vi "Sender.vi"() -> ()   [LabVIEW 2014]
uses:
  Global 1.vi
panel:
  out "Waveform Chart":dbl(graph)
  in  "Saving":bool
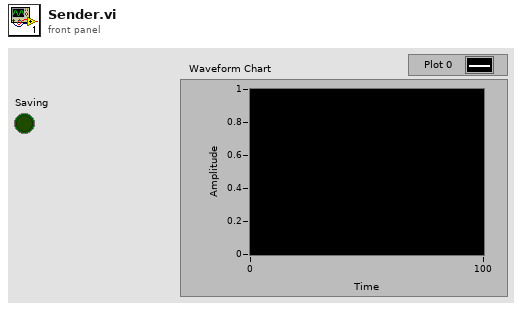
[diagram p1: front panel]
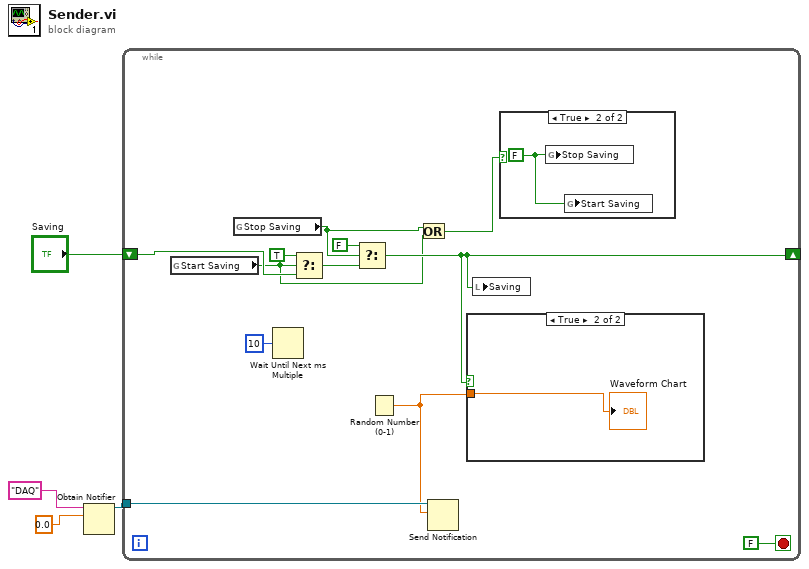
[diagram p0: block diagram]
diagram:
  n1 = Obtain Notifier(name (unnamed)="DAQ", notification data type=0.0) -> (notifier out=w3:refnum<notifier>)  [unwired: 2 in, 2 out]
  n2 = while {
    tunnel: w3 -> [w15]
    shift-right: [w8] -> _
    shift-left: "Saving" -> [w10]
    stop <- FALSE stop-if-true
    n3 = global read "Global 1.vi" "Start Saving"() -> (w6:bool)
    n4 = global read "Global 1.vi" "Stop Saving"() -> (w7:bool)
    n5 = Wait Until Next ms Multiple(millisecond multiple=u32 10) -> ()  [unwired: 1 out]
    n6 = Select(t=TRUE, s=w6, f=w10) -> (s? t:f=w12:bool)
    n7 = Select(t=FALSE, s=w7, f=w12) -> (s? t:f=w8:bool)
    n8 = Random Number (0-1)() -> (number: 0 to 1=w14:dbl)
    n9 = Or(x=w7, y=w6) -> (x .or. y?=w5:bool)
    n10 = Send Notification(notification=w14, notifier=w15) -> ()  [unwired: 1 in, 2 out]
    n11 = case shown="True" w8 {
      tunnel: w14 -> [_ w18]
      frame False {
      }
      frame True {
        "Waveform Chart" <- w18
      }
    }
    n12 = local write "Saving"(w8) -> ()
    n13 = case shown="True" w5 {
      frame False {
      }
      frame True {
        w17 = FALSE
        n14 = global write "Global 1.vi" "Stop Saving"(w17) -> ()
        n15 = global write "Global 1.vi" "Start Saving"(w17) -> ()
      }
    }
  }
